vi "List Config Types.vi"() -> (2 "Config types":string[](array[string]))   [LabVIEW 2019, in "Attribute.Config.lvclass"]
doc: "JKI State Machine Objects (SMO) 1.3.0.56\nJKI - JKI\nCopyright (c) 2017, JKI"
uses:
  Attribute.Config.lvclass
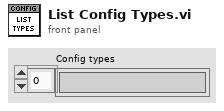
[diagram p1: front panel]
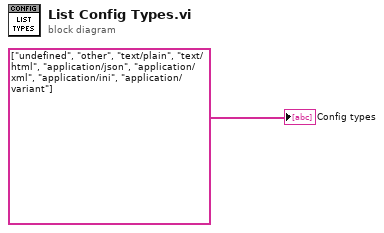
[diagram p0: block diagram]
diagram:
  "Config types" <- string[] ["undefined", "other", "text/plain", "text/html", "application/json", "application/xml", "application/ini", "application/variant"] ("Config types 2")
